vi "Manual Shooter Mode.vi"() -> (1 "Right Output":dbl, 3 "Left Output":dbl)   [LabVIEW 2015]
uses:
  Robot Global Data.vi
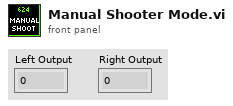
[diagram p1: front panel]
types:
  T1 = typedef "Dashboard Control Data.ctl" = cluster{"Auton Loops":dbl, "Shooter Presets":T2}
  T2 = typedef "Shooter Presets.ctl" = cluster{"Batter Shot":T3, "Low Bar Curve Shot":T3, "Deep Middle Shot":T3, "Manual Shot":T3}
  T3 = typedef "Shot Presets.ctl" = cluster{"Left Wheel RPM":dbl, "Right Wheel RPM":dbl}
  T4 = typedef "Manual Shoot.ctl" = cluster{"Spin Wheels":bool, "Fire":bool}
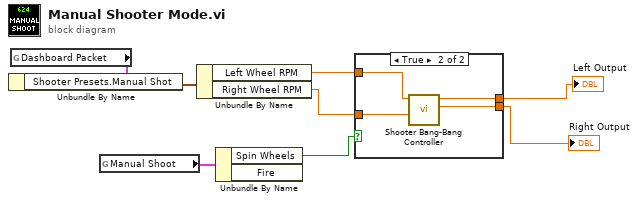
[diagram p0: block diagram]
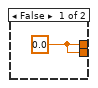
[diagram p2: hidden frame]
diagram:
  n1 = global read "Robot Global Data.vi" "Dashboard Packet"() -> (w7:T1)
  n2 = Unbundle By Name(w7) -> ("Shooter Presets.Manual Shot"=w6:T3)
  n3 = global read "Robot Global Data.vi" "Manual Shoot"() -> (w8:T4)
  n4 = Unbundle By Name(w6) -> ("Left Wheel RPM"=w4:dbl, "Right Wheel RPM"=w3:dbl)
  n5 = Unbundle By Name(w8) -> ("Spin Wheels"=w5:bool)  [unwired: 1 out]
  n6 = case shown="True" w5 {
    tunnel: w4 -> [_ w13]
    tunnel: w3 -> [_ w12]
    tunnel: [w9 w11] -> w1
    tunnel: [w9 w10] -> w2
    frame False {
      w9 = 0.0 ("Left Output Power")
    }
    frame True {
      n7 = call "Shooter Bang-Bang Controller.vi"("Right Target RPM"=w12, "Left Target RPM"=w13) -> ("Right Output Power"=w10:dbl, "Left Output Power"=w11:dbl)  [unwired: 8 in]
    }
  }
  "Left Output" <- w1
  "Right Output" <- w2
